vi "Untitled5.vi"() -> ()   [LabVIEW 2024]
uses:
  CANopen Master/CANopen Master.lvclass
  <vilib>/ProgressBar/Progress Bar Dialog.lvclass
  EDS-File-Viewer/Electronic Datasheet/Electronic Datasheet.lvclass
  HAL/Source/Communicator/Communicator.lvclass
  EDS-File-Viewer/Core/OD Entry/OD Entry.lvclass
  EDS-File-Viewer/Core/OD Sub-Entry/OD Sub-Entry.lvclass
panel:
  out "Success":bool[](array[boolean])
  out "Objects List":string[](array[string])
  out "Values":variant[](array[variant])
  in  "Actual Values Button":bool
  out "Uploaded":variant
  out "MSG Log":string
  in  "Discover Button":bool
  out "Success? DL":bool
  in  "Value":u16
  in  "Multiplexer DL":cluster{"Index":u16, "Sub-Index":u8} {"Index" format="%.0x"}
  in  "Download Button":bool
  in  "Node-ID DL":u8
  out "Available Nodes":map{u8, u8}(c390)
  out "Success? UL":bool
  out "Data UL":u8[](array[numeric]) format="%.0x"
  in  "Node-ID UPL":u8
  in  "Multiplexer":cluster{"Index":u16, "Sub-Index":u8} {"Index" format="%.0x"}
  in  "Upload Button":bool
  out "Emergency?":bool[](array[boolean])
  out "Nodes":u8[](array[numeric])
  in  "stop":bool
  out "Timed Outs?":bool[](array[boolean])
  out "Node-IDs":u8[](array[numeric])
  out "error out":errorcluster
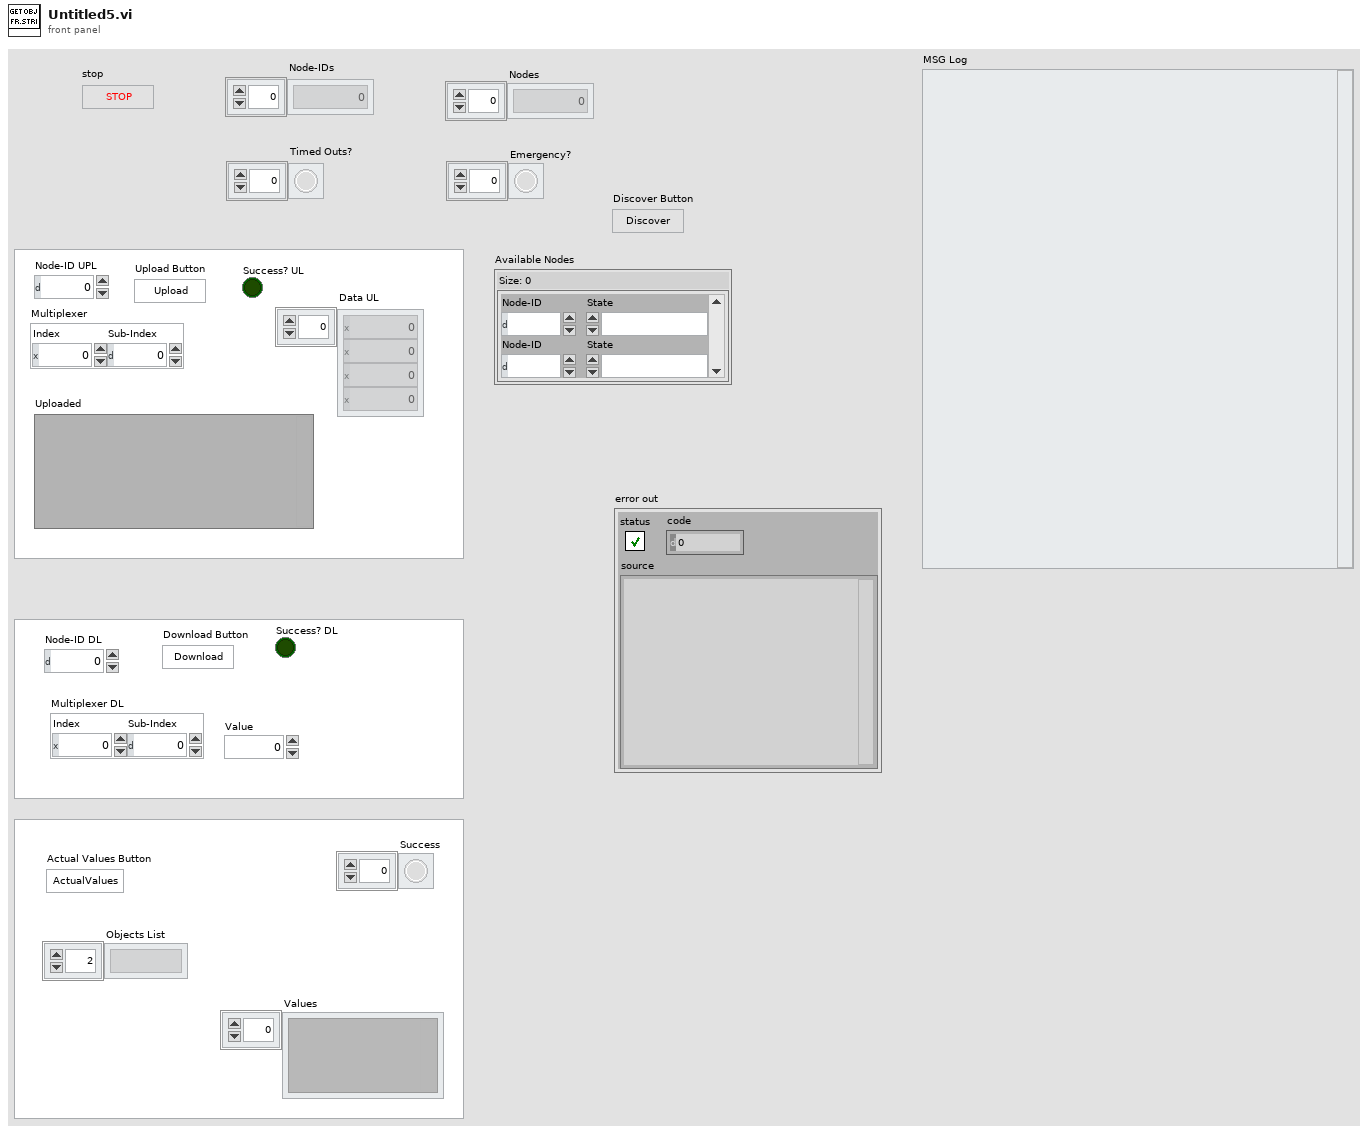
[diagram p1: front panel]
types:
  T1 = cluster{"Stop CAN Task":refnum<user-event>, "Msg Received":refnum<user-event>, "CAN Task Error":refnum<user-event>, "Node Discovered":refnum<user-event>}
  T2 = cluster{"Msg Received":refnum<user-event>, "CAN Task Error":refnum<user-event>, "Node Discovered":refnum<user-event>}
  T3 = typedef "EDS.lvlib/Data Type.ctl" = u16
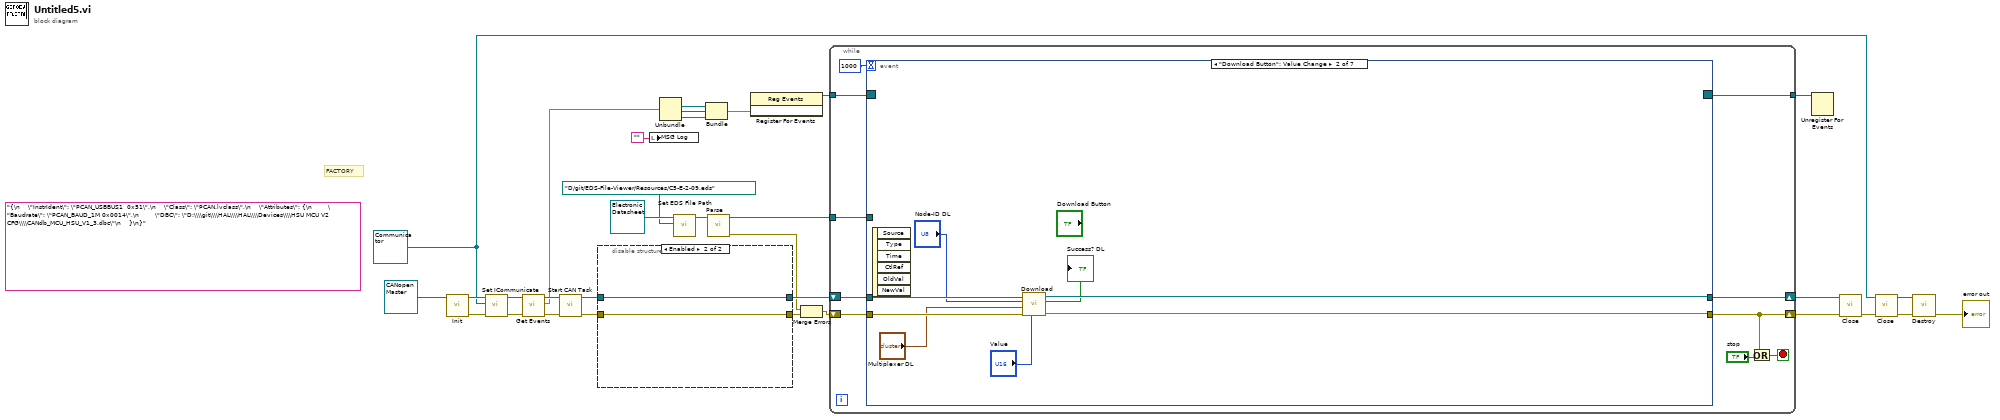
[diagram p0: block diagram]
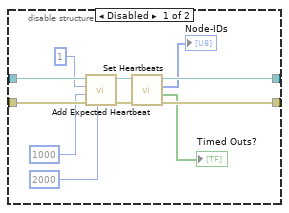
[diagram p2: hidden frame]
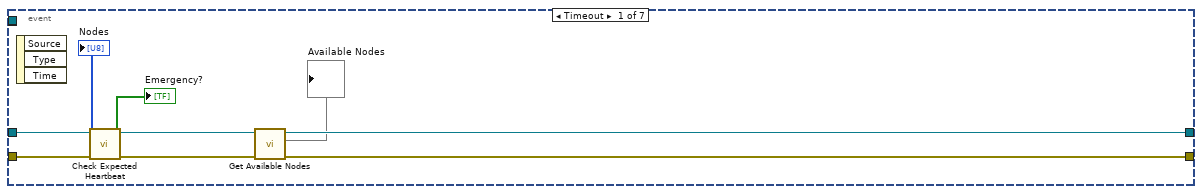
[diagram p3: hidden frame]
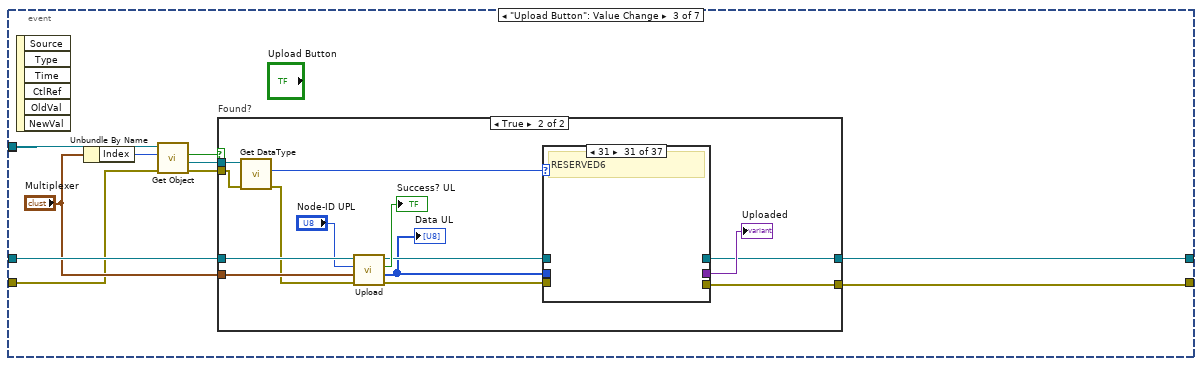
[diagram p4: hidden frame]
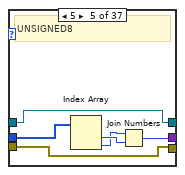
[diagram p10: hidden frame]
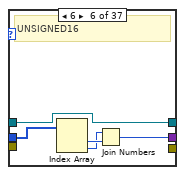
[diagram p11: hidden frame]
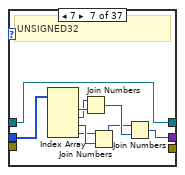
[diagram p12: hidden frame]
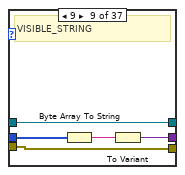
[diagram p14: hidden frame]
diagram:
  w4 = refnum<class "Communicator.lvclass"> refnum ("Communicator")
  (unwired) "{\n    \"InstrIdent\": \"PCAN_USBBUS1  0x51\",\n    \"Class\": \"PCAN.lvclass\",\n    \"Attributes\": {\n        \"Baudrate\": \"PCAN_BAUD_1M 0x0014\",\n        \"DBC\": \"D:\\\\git\\\\HAL\\\\HAL\\\\Devices\\\\HSU MCU V2 CFG\\\\CANdb_MCU_HSU_V1_3.dbc\"\n    }\n}" ("<JSON>CFG")
  # "FACTORY"
  n1 = call "Init.vi"("CANopen Master in"=refnum<class "CANopen Master.lvclass"> refnum ("CANopen Master.lvlib:CANopen Master")) -> ("error out"=w27:errorcluster, "CANopen Master out"=w28:refnum<class "CANopen Master.lvclass">)  [unwired: 9 in]
  n2 = call "Set ICommunicate.vi"("ICommunicate"=w4, "CANopen Master in"=w28) -> ("CANopen Master out"=w11:refnum<class "CANopen Master.lvclass">)  [unwired: 9 in]
  n3 = call "Get Events.vi"("CANopen Master in"=w11) -> ("Events"=w9:T1, "CANopen Master out"=w10:refnum<class "CANopen Master.lvclass">)  [unwired: 9 in]
  n4 = call "Start CAN Task.vi"("error in"=w27, "CANopen Master in"=w10) -> ("error out"=w15:errorcluster, "CANopen Master out"=w14:refnum<class "CANopen Master.lvclass">)  [unwired: 8 in]
  n5 = disable-structure shown="Enabled" {
    disable-tunnel: w15 -> [w41 w42]
    disable-tunnel: w14 -> [w40 w43]
    disable-tunnel: [w39 w43] -> w26
    disable-tunnel: [w38 w42] -> w25
    frame Disabled {
      n6 = call "Add Expected Heartbeat.vi"("Timeout"=u16 2000, "error in"=w41, "Period"=u16 1000, "Node-ID"=u8 1, "CANopen Master in"=w40) -> ("error out"=w34:errorcluster, "CANopen Master out"=w33:refnum<class "CANopen Master.lvclass">)  [unwired: 5 in]
      n7 = call "Set Heartbeats.vi"("error in"=w34, "CANopen Master in"=w33) -> ("error out"=w38:errorcluster, "Timed Outs?"=→"Timed Outs?":bool[], "Node-IDs"=→"Node-IDs":u8[], "CANopen Master out"=w39:refnum<class "CANopen Master.lvclass">)  [unwired: 6 in]
    }
    frame Enabled {
    }
  }
  n8 = local write "MSG Log"("") -> ()
  n9 = Unbundle(w9) -> ("Msg Received"=w7:refnum<user-event>, "CAN Task Error"=w6:refnum<user-event>, "Node Discovered"=w5:refnum<user-event>)  [unwired: 1 out]
  n10 = call "Set EDS File Path.vi"("EDS File Path"=path "D:/git/EDS-File-Viewer/Resources/C5-E-2-09.eds", "reference in"=refnum<class "Electronic Datasheet.lvclass"> refnum ("Electronic Datasheet.lvlib:Electronic Datasheet")) -> ("reference out"=w19:refnum<class "Electronic Datasheet.lvclass">)  [unwired: 8 in, 1 out]
  n11 = Bundle("Msg Received"=w7, "CAN Task Error"=w6, "Node Discovered"=w5) -> (w8:T2)  [unwired: 1 in]
  n12 = call "Parse.vi"("reference in"=w19) -> ("error out"=w17:errorcluster, "reference out"=w16:refnum<class "Electronic Datasheet.lvclass">)  [unwired: 9 in]
  n13 = register-events(w8) -> (reference out=w13:refnum<event-registration>)  [unwired: 2 in, 1 out]
  n14 = Merge Errors(w17, w25) -> (w18:errorcluster)
  n15 = while {
    shift-right: [w50] -> w23
    shift-left: w26 -> [w52]
    shift-right: [w49] -> w24
    shift-left: w18 -> [w51]
    tunnel: w16 -> [w46]
    tunnel: w13 -> [w45]
    tunnel: [w44] -> w12
    stop <- w48 stop-if-true
    n16 = event shown="[1] \"Download Button\": Value Change" {
      selector: w45 -> [_ _ _ _ _ _ _]
      dyn-events: [_ _ _ _ _ _ _] -> w44
      timeout: 1000 -> [_ _ _ _ _ _ _]
      tunnel: w52 -> [w60 w68 w79 w135 w236 w243 w251]
      tunnel: w51 -> [w61 w69 w72 w136 w237 w244 w252]
      tunnel: [w59 w67 w76 w127 w237 w244 w250] -> w49
      tunnel: [w55 w66 w75 w123 w236 w243 w249] -> w50
      tunnel: w46 -> [_ _ w78 w124 _ _ _]
      tunnel: [_ _ w78 _ _ _ _] -> _
      event Timeout {
        n17 = event-data() -> ()  [unwired: 1 in, 3 out]
        n18 = call "Check Expected Heartbeat.vi"("error in"=w61, "CANopen Master in"=w60) -> ("error out"=w59:errorcluster, "Emergency?"=→"Emergency?":bool[], "Nodes"=→"Nodes":u8[], "CANopen Master out"=w58:refnum<class "CANopen Master.lvclass">)  [unwired: 6 in]
        n19 = call "Get Available Nodes.vi"("CANopen Master in"=w58) -> ("Nodes"=→"Available Nodes":map{u8, u8}, "CANopen Master out"=w55:refnum<class "CANopen Master.lvclass">)  [unwired: 8 in, 1 out]
      }
      event "Download Button": Value Change {
        n20 = event-data() -> ()  [unwired: 1 in, 6 out]
        n21 = call "Download.vi"("Value"="Value", "error in"=w69, "Multiplexer"="Multiplexer DL", "Node-ID"="Node-ID DL", "CANopen Master in"=w68) -> ("error out"=w67:errorcluster, "Success?"=→"Success? DL":bool, "CANopen Master out"=w66:refnum<class "CANopen Master.lvclass">)  [unwired: 4 in]
      }
      event "Upload Button": Value Change {
        n22 = event-data() -> ()  [unwired: 1 in, 6 out]
        n23 = Unbundle By Name("Multiplexer") -> ("Index"=w74:u16)
        n24 = call "Get Object.vi"("error in"=w72, "Index"=w74, "reference in"=w78) -> ("error out"=w71:errorcluster, "OD Entry"=w73:refnum<class "OD Entry.lvclass">, "Found?"=w70:bool)  [unwired: 5 in, 1 out]
        n25 = case "Found?" shown="True" w70 {
          tunnel: w79 -> [w81 w95]
          tunnel: "Multiplexer" -> [_ w94]
          tunnel: [w80 w87] -> w76
          tunnel: [w81 w86] -> w75
          tunnel: w73 -> [_ w85]
          tunnel: w71 -> [w80 w84]
          frame False {
          }
          frame True {
            n26 = call "Get DataType.vi"("Error In"=w84, "reference in"=w85) -> ("Error Out"=w82:errorcluster, "DataType"=w92:u16)  [unwired: 7 in, 1 out]
            n27 = call "Upload.vi"("error in"=w82, "Multiplexer"=w94, "Node-ID"="Node-ID UPL", "CANopen Master in"=w95) -> ("error out"=w90:errorcluster, "Value"=w89:u8[], "Success?"=→"Success? UL":bool, "CANopen Master out"=w91:refnum<class "CANopen Master.lvclass">)  [unwired: 4 in]
            "Data UL" <- w89
            n28 = case shown="31" w92 {
              tunnel: w91 -> [_ _ _ _ w100 w102 w107 _ w117 _ _ _ _ _ _ _ _ _ _ _ _ _ _ _ _ _ _ _ _ _ _ _ _ _ _ _ w122]
              tunnel: w90 -> [_ _ _ _ w96 _ _ _ w118 _ _ _ _ _ _ _ _ _ _ _ _ _ _ _ _ _ _ _ _ _ _ _ _ _ _ _ w121]
              tunnel: w89 -> [_ _ _ _ w101 w106 w115 _ w120 _ _ _ _ _ _ _ _ _ _ _ _ _ _ _ _ _ _ _ _ _ _ _ _ _ _ _ _]
              tunnel: [_ _ _ _ w97 w103 w108 _ w116 _ _ _ _ _ _ _ _ _ _ _ _ _ _ _ _ _ _ _ _ _ _ _ _ _ _ _ _] -> w88
              tunnel: [_ _ _ _ w96 _ _ _ w118 _ _ _ _ _ _ _ _ _ _ _ _ _ _ _ _ _ _ _ _ _ _ _ _ _ _ _ w121] -> w87
              tunnel: [_ _ _ _ w100 w102 w107 _ w117 _ _ _ _ _ _ _ _ _ _ _ _ _ _ _ _ _ _ _ _ _ _ _ _ _ _ _ w122] -> w86
              frame 1 {
                # "BOOLEAN"
              }
              frame 2 {
                # "INTEGER8"
              }
              frame 3 {
                # "INTEGER16"
              }
              frame 4 {
                # "INTEGER32"
              }
              frame 5 {
                # "UNSIGNED8"
                n29 = Index Array(array=w101) -> (element #1=w99:u8, element #2=w98:u8)  [unwired: 2 in]
                n30 = Join Numbers(hi=w98, lo=w99) -> ((hi.lo)=w97:u16)
              }
              frame 6 {
                # "UNSIGNED16"
                n31 = Index Array(array=w106) -> (element #1=w105:u8, element #2=w104:u8)  [unwired: 2 in]
                n32 = Join Numbers(hi=w104, lo=w105) -> ((hi.lo)=w103:u16)
              }
              frame 7 {
                # "UNSIGNED32"
                n33 = Index Array(array=w115) -> (element #1=w114:u8, element #2=w113:u8, element #3=w112:u8, element #4=w111:u8)  [unwired: 4 in]
                n34 = Join Numbers(hi=w113, lo=w114) -> ((hi.lo)=w110:u16)
                n35 = Join Numbers(hi=w111, lo=w112) -> ((hi.lo)=w109:u16)
                n36 = Join Numbers(hi=w109, lo=w110) -> ((hi.lo)=w108:u32)
              }
              frame 8 {
                # "REAL32"
              }
              frame 9 {
                # "VISIBLE_STRING"
                n37 = Byte Array To String(unsigned byte array=w120) -> (string=w119:string)
                n38 = To Variant(anything=w119) -> (Variant=w116:variant)
              }
              frame 10 {
                # "OCTET_STRING"
              }
              frame 11 {
                # "UNICODE_STRING"
              }
              frame 12 {
                # "TIME_OF_DAY"
              }
              frame 13 {
                # "TIME_DIFFERENCE"
              }
              frame 14 {
                # "RESERVED1"
              }
              frame 15 {
                # "DOMAIN"
              }
              frame 16 {
                # "INTEGER24"
              }
              frame 17 {
                # "REAL64"
              }
              frame 18 {
                # "INTEGER40"
              }
              frame 19 {
                # "INTEGER48"
              }
              frame 20 {
                # "INTEGER56"
              }
              frame 21 {
                # "INTEGER64"
              }
              frame 22 {
                # "UNSIGNED24"
              }
              frame 23 {
                # "RESERVED2"
              }
              frame 24 {
                # "UNSIGNED40"
              }
              frame 25 {
                # "UNSIGNED48"
              }
              frame 26 {
                # "UNSIGNED56"
              }
              frame 27 {
                # "UNSIGNED64"
              }
              frame 28 {
                # "RESERVED3"
              }
              frame 29 {
                # "RESERVED4"
              }
              frame 30 {
                # "RESERVED5"
              }
              frame 31 {
                # "RESERVED6"
              }
              frame 32 {
                # "PDO_COMMUNICATION_PARAMETER"
              }
              frame 33 {
                # "PDO_MAPPING"
              }
              frame 34 {
                # "SDO_PARAMETER"
              }
              frame 35 {
                # "IDENTITY"
              }
              frame 36 {
                # "RESERVED7"
              }
              frame Default {
                # "INVALID"
              }
            }
            "Uploaded" <- w88
          }
        }
      }
      event "Actual Values Button": Value Change {
        n39 = event-data() -> ()  [unwired: 1 in, 6 out]
        n40 = call "Get Communication Specific Objects.vi"("error in"=w136, "Electronic Datasheet"=w124) -> ("error out"=w129:errorcluster, "Entries"=w126:refnum<class "OD Entry.lvclass">[])  [unwired: 7 in, 1 out]
        n41 = local read "Node-ID UPL"() -> (w128:u8)
        n42 = Array Size(array=w126) -> (size(s)=w132:i32)
        n43 = call <vilib>:"Launch Progress Bar.vi"("Main Title (\"Working...\")"="Uploading Actual Values" ("Main Title (\"Working...\")"), "Total Count"=w132) -> ("Progress Bar Dialog"=w134:refnum<class "Progress Bar Dialog.lvclass">)  [unwired: 8 in, 1 out]
        n44 = for {
          tunnel: w126 -> [w142] mode=indexing
          shift-right: [w151] -> w133
          shift-left: w134 -> [w152]
          tunnel: [w154] -> w130 mode=concatenating
          shift-right: [w150] -> w123
          shift-left: w135 -> [w155]
          tunnel: w128 -> [w149]
          shift-right: [w148] -> w127
          shift-left: w129 -> [w138]
          tunnel: [w143] -> w125 mode=concatenating
          n45 = call "Get Index.vi"("Error In"=w138, "reference in"=w142) -> ("Error Out"=w137:errorcluster, "Index"=w141:u16, "reference out"=w139:refnum<class "OD Entry.lvclass">)  [unwired: 7 in]
          n46 = call "Get All Sub-Entries.vi"("Error In"=w137, "reference in"=w139) -> ("Error Out"=w153:errorcluster, "Indices"=w146:u8[], "Sub-Entries"=w145:refnum<class "OD Sub-Entry.lvclass">[], "reference out"=w144:refnum<class "OD Entry.lvclass">)  [unwired: 6 in]
          n47 = Number To Hexadecimal String(2:w141) -> (0:w140:string)  [unwired: 1 in]
          n48 = call <vilib>:"Increment Progress Bar.vi"("Step Name (\"\")"=w140, "Progress Bar Dialog in"=w152) -> ("Progress Bar Dialog out"=w151:refnum<class "Progress Bar Dialog.lvclass">)  [unwired: 7 in, 2 out]
          n49 = Array Size(array=w145) -> (size(s)=w147:i32)
          n50 = case "Index has Sub-Entries?" shown="0" w147 {
            tunnel: w155 -> [w171 w200]
            tunnel: [w166 w194] -> w154
            tunnel: w153 -> [w161 w196]
            tunnel: w146 -> [_ w192]
            tunnel: [w164 w199] -> w150
            tunnel: w149 -> [w167 w198]
            tunnel: [w165 w195] -> w148
            tunnel: w145 -> [_ w193]
            tunnel: w144 -> [w159 _]
            tunnel: [w157 w191] -> w143
            tunnel: w140 -> [w156 _]
            frame 0 {
              n51 = Bundle(w156, "") -> (w162:cluster{string, string})  [unwired: 1 in]
              n52 = call "Upload from String.vi"("error in"=w161, "Multiplexer"=w162, "Node-ID"=w167, "CANopen Master in"=w171) -> ("error out"=w160:errorcluster, "Value"=w170:u8[], "Success?"=w158:bool, "CANopen Master out"=w164:refnum<class "CANopen Master.lvclass">)  [unwired: 4 in]
              n53 = call "Get DataType.vi"("Error In"=w160, "reference in"=w159) -> ("Error Out"=w165:errorcluster, "DataType"=w168:u16)  [unwired: 7 in, 1 out]
              n54 = case shown="7" w168 {
                tunnel: w170 -> [_ _ _ _ w175 w179 w187 _ w190 _ _ _ _ _ _ _ _ _ _ _ _ _ _ _ _ _ _ _ _ _ _ _ _ _ _ _ _]
                tunnel: [_ _ _ _ w172 w176 w180 _ w188 _ _ _ _ _ _ _ _ _ _ _ _ _ _ _ _ _ _ _ _ _ _ _ _ _ _ _ _] -> w169
                frame 1 {
                  # "BOOLEAN"
                }
                frame 2 {
                  # "INTEGER8"
                }
                frame 3 {
                  # "INTEGER16"
                }
                frame 4 {
                  # "INTEGER32"
                }
                frame 5 {
                  # "UNSIGNED8"
                  n55 = Index Array(array=w175) -> (element #1=w174:u8, element #2=w173:u8)  [unwired: 2 in]
                  n56 = Join Numbers(hi=w173, lo=w174) -> ((hi.lo)=w172:u16)
                }
                frame 6 {
                  # "UNSIGNED16"
                  n57 = Index Array(array=w179) -> (element #1=w178:u8, element #2=w177:u8)  [unwired: 2 in]
                  n58 = Join Numbers(hi=w177, lo=w178) -> ((hi.lo)=w176:u16)
                }
                frame 7 {
                  # "UNSIGNED32"
                  n59 = Index Array(array=w187) -> (element #1=w186:u8, element #2=w185:u8, element #3=w184:u8, element #4=w183:u8)  [unwired: 4 in]
                  n60 = Join Numbers(hi=w185, lo=w186) -> ((hi.lo)=w182:u16)
                  n61 = Join Numbers(hi=w183, lo=w184) -> ((hi.lo)=w181:u16)
                  n62 = Join Numbers(hi=w181, lo=w182) -> ((hi.lo)=w180:u32)
                }
                frame 8 {
                  # "REAL32"
                }
                frame 9 {
                  # "VISIBLE_STRING"
                  n63 = Byte Array To String(unsigned byte array=w190) -> (string=w189:string)
                  n64 = To Variant(anything=w189) -> (Variant=w188:variant)
                }
                frame 10 {
                  # "OCTET_STRING"
                }
                frame 11 {
                  # "UNICODE_STRING"
                }
                frame 12 {
                  # "TIME_OF_DAY"
                }
                frame 13 {
                  # "TIME_DIFFERENCE"
                }
                frame 14 {
                  # "RESERVED1"
                }
                frame 15 {
                  # "DOMAIN"
                }
                frame 16 {
                  # "INTEGER24"
                }
                frame 17 {
                  # "REAL64"
                }
                frame 18 {
                  # "INTEGER40"
                }
                frame 19 {
                  # "INTEGER48"
                }
                frame 20 {
                  # "INTEGER56"
                }
                frame 21 {
                  # "INTEGER64"
                }
                frame 22 {
                  # "UNSIGNED24"
                }
                frame 23 {
                  # "RESERVED2"
                }
                frame 24 {
                  # "UNSIGNED40"
                }
                frame 25 {
                  # "UNSIGNED48"
                }
                frame 26 {
                  # "UNSIGNED56"
                }
                frame 27 {
                  # "UNSIGNED64"
                }
                frame 28 {
                  # "RESERVED3"
                }
                frame 29 {
                  # "RESERVED4"
                }
                frame 30 {
                  # "RESERVED5"
                }
                frame 31 {
                  # "RESERVED6"
                }
                frame 32 {
                  # "PDO_COMMUNICATION_PARAMETER"
                }
                frame 33 {
                  # "PDO_MAPPING"
                }
                frame 34 {
                  # "SDO_PARAMETER"
                }
                frame 35 {
                  # "IDENTITY"
                }
                frame 36 {
                  # "RESERVED7"
                }
                frame Default {
                  # "INVALID"
                }
              }
              n65 = Build Array(w158) -> (w157:bool[])
              n66 = Build Array(w169) -> (w166:variant[])
            }
            frame Default {
              n67 = for {
                shift-right: [w215] -> w199
                shift-left: w200 -> [w216]
                tunnel: w198 -> [w214]
                tunnel: [w213] -> w197
                shift-right: [w209] -> w195
                shift-left: w196 -> [w211]
                tunnel: w193 -> [w207] mode=indexing
                tunnel: [w205] -> w194 mode=indexing
                tunnel: w192 -> [w202] mode=indexing
                tunnel: [w201] -> w191 mode=indexing
                n68 = Format Into String(format string="%d", w202) -> (resulting string=w203:string)  [unwired: 2 in, 1 out]
                n69 = Bundle(w213, w203) -> (w212:cluster{void, string})  [unwired: 1 in]
                n70 = call "Upload from String.vi"("error in"=w211, "Multiplexer"=w212, "Node-ID"=w214, "CANopen Master in"=w216) -> ("error out"=w210:errorcluster, "Value"=w206:u8[], "Success?"=w201:bool, "CANopen Master out"=w215:refnum<class "CANopen Master.lvclass">)  [unwired: 4 in]
                n71 = call "Get DataType+.vi"("Error In"=w210, "reference in"=w207) -> ("Error Out"=w209:errorcluster, "DataType"=w208:T3)  [unwired: 6 in, 2 out]
                n72 = case shown="7" w208 {
                  tunnel: w206 -> [_ _ _ _ w220 w224 w232 _ w235 _ _ _ _ _ _ _ _ _ _ _ _ _ _ _ _ _ _ _ _ _ _ _ _ _ _ _ _]
                  tunnel: [_ _ _ _ w217 w221 w225 _ w233 _ _ _ _ _ _ _ _ _ _ _ _ _ _ _ _ _ _ _ _ _ _ _ _ _ _ _ _] -> w205
                  frame 1 {
                    # "BOOLEAN"
                  }
                  frame 2 {
                    # "INTEGER8"
                  }
                  frame 3 {
                    # "INTEGER16"
                  }
                  frame 4 {
                    # "INTEGER32"
                  }
                  frame 5 {
                    # "UNSIGNED8"
                    n73 = Index Array(array=w220) -> (element #1=w219:u8, element #2=w218:u8)  [unwired: 2 in]
                    n74 = Join Numbers(hi=w218, lo=w219) -> ((hi.lo)=w217:u16)
                  }
                  frame 6 {
                    # "UNSIGNED16"
                    n75 = Index Array(array=w224) -> (element #1=w223:u8, element #2=w222:u8)  [unwired: 2 in]
                    n76 = Join Numbers(hi=w222, lo=w223) -> ((hi.lo)=w221:u16)
                  }
                  frame 7 {
                    # "UNSIGNED32"
                    n77 = Index Array(array=w232) -> (element #1=w231:u8, element #2=w230:u8, element #3=w229:u8, element #4=w228:u8)  [unwired: 4 in]
                    n78 = Join Numbers(hi=w230, lo=w231) -> ((hi.lo)=w227:u16)
                    n79 = Join Numbers(hi=w228, lo=w229) -> ((hi.lo)=w226:u16)
                    n80 = Join Numbers(hi=w226, lo=w227) -> ((hi.lo)=w225:u32)
                  }
                  frame 8 {
                    # "REAL32"
                  }
                  frame 9 {
                    # "VISIBLE_STRING"
                    n81 = Byte Array To String(unsigned byte array=w235) -> (string=w234:string)
                    n82 = To Variant(anything=w234) -> (Variant=w233:variant)
                  }
                  frame 10 {
                    # "OCTET_STRING"
                  }
                  frame 11 {
                    # "UNICODE_STRING"
                  }
                  frame 12 {
                    # "TIME_OF_DAY"
                  }
                  frame 13 {
                    # "TIME_DIFFERENCE"
                  }
                  frame 14 {
                    # "RESERVED1"
                  }
                  frame 15 {
                    # "DOMAIN"
                  }
                  frame 16 {
                    # "INTEGER24"
                  }
                  frame 17 {
                    # "REAL64"
                  }
                  frame 18 {
                    # "INTEGER40"
                  }
                  frame 19 {
                    # "INTEGER48"
                  }
                  frame 20 {
                    # "INTEGER56"
                  }
                  frame 21 {
                    # "INTEGER64"
                  }
                  frame 22 {
                    # "UNSIGNED24"
                  }
                  frame 23 {
                    # "RESERVED2"
                  }
                  frame 24 {
                    # "UNSIGNED40"
                  }
                  frame 25 {
                    # "UNSIGNED48"
                  }
                  frame 26 {
                    # "UNSIGNED56"
                  }
                  frame 27 {
                    # "UNSIGNED64"
                  }
                  frame 28 {
                    # "RESERVED3"
                  }
                  frame 29 {
                    # "RESERVED4"
                  }
                  frame 30 {
                    # "RESERVED5"
                  }
                  frame 31 {
                    # "RESERVED6"
                  }
                  frame 32 {
                    # "PDO_COMMUNICATION_PARAMETER"
                  }
                  frame 33 {
                    # "PDO_MAPPING"
                  }
                  frame 34 {
                    # "SDO_PARAMETER"
                  }
                  frame 35 {
                    # "IDENTITY"
                  }
                  frame 36 {
                    # "RESERVED7"
                  }
                  frame Default {
                    # "INVALID"
                  }
                }
              }
            }
          }
        }
        "Values" <- w130
        "Success" <- w125
        n83 = call <vilib>:"Close Progress Bar.vi"("Progress Bar Dialog"=w133) -> ()  [unwired: 10 in, 1 out]
      }
      event User Event {
        n84 = event-data() -> ("status"=w241:bool, "code"=w240:i32, "source"=w239:string)  [unwired: 1 in]
        n85 = Bundle By Name(cluster=errorcluster {"status"=FALSE, "code"=0, "source"=""} ("error constant"), "status"=w241, "code"=w240, "source"=w239) -> (w238:errorcluster)
        n86 = call <vilib>:"Simple Error Handler.vi"("error in (no error)"=w238) -> ()  [unwired: 4 in, 5 out]
      }
      event User Event {
        n87 = event-data() -> ("Message"=w245:string)  [unwired: 1 in, 4 out]
        n88 = local read "MSG Log"() -> (w247:string)
        n89 = Concatenate Strings(w245, "\r", w247) -> (→"MSG Log":string)
      }
      event "Discover Button": Value Change {
        n90 = event-data() -> ()  [unwired: 1 in, 6 out]
        n91 = call "Discover Nodes.vi"("error in"=w252, "CANopen Master in"=w251) -> ("error out"=w250:errorcluster, "CANopen Master out"=w249:refnum<class "CANopen Master.lvclass">)  [unwired: 8 in]
      }
    }
    n92 = Or(x=w49, y="stop") -> (x .or. y?=w48:bool)
  }
  n93 = Unregister For Events(event registration refnum=w12) -> ()  [unwired: 1 in, 1 out]
  n94 = call "Close.vi"("error in"=w24, "CANopen Master in"=w23) -> ("error out"=w29:errorcluster)  [unwired: 8 in, 1 out]
  n95 = call-dynamic "Close.vi"("Error In"=w29, "Communicator in"=w4) -> ("Error Out"=w2:errorcluster, "Communicator out"=w3:refnum<class "Communicator.lvclass">)  [unwired: 8 in]
  n96 = call-dynamic "Destroy.vi"("Error In"=w2, "Communicator in"=w3) -> ("Error Out"=→"error out":errorcluster)  [unwired: 8 in, 1 out]
